vi "排气扇参数配置.vi"() -> ()   [LabVIEW 2016, in "环境动力监测库.lvlib"]
panel:
  in  "功能启用":bool
  in  "排气扇关闭温度":dbl=60.0 caption="关闭温度" format="%#_2f ℃"
  in  "排气扇开启温度":dbl=60.0 caption="开启温度" format="%#.2f ℃"
  # "排气扇参数配置"
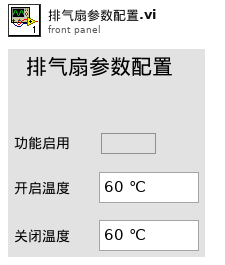
[diagram p1: front panel]
types:
  T1 = cluster{"功能启用":bool, "排气扇开启温度":dbl, "排气扇关闭温度":dbl}
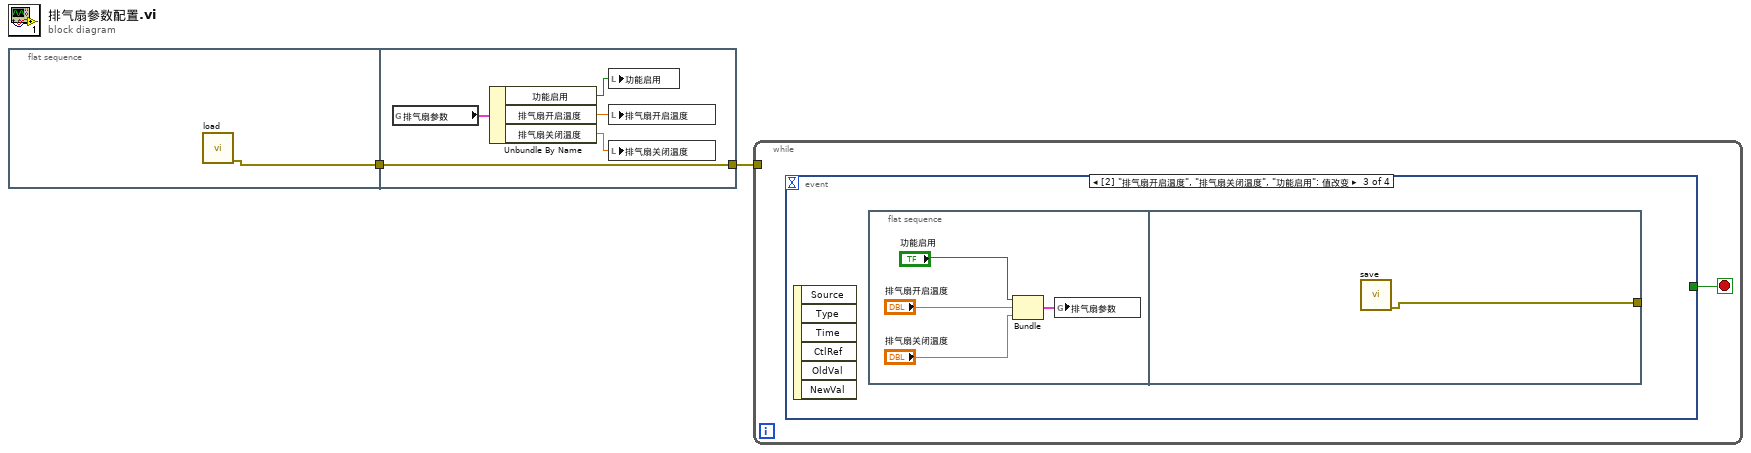
[diagram p0: block diagram]
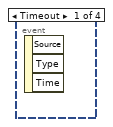
[diagram p2: hidden frame]
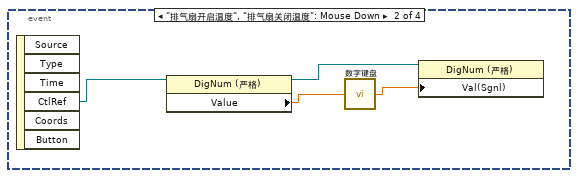
[diagram p3: hidden frame]
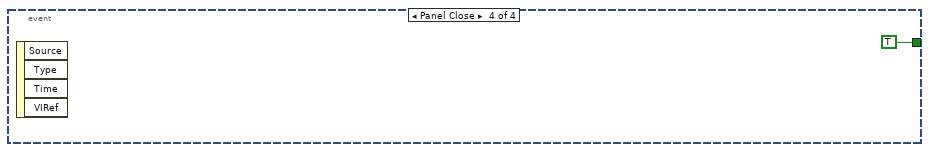
[diagram p4: hidden frame]
diagram:
  n1 = flat-sequence {
    tunnel: [w3] -> w2
    tunnel: [w8] -> w1
    tunnel: w2 -> [w8]
    frame #0 {
      n2 = call "load.vi"() -> ("error out"=w3:errorcluster)  [unwired: 11 in]
    }
    frame #1 {
      n3 = global read "断电保存全局变量.vi" "排气扇参数"() -> (w7:T1)
      n4 = Unbundle By Name(w7) -> ("功能启用"=w6:bool, "排气扇开启温度"=w5:dbl, "排气扇关闭温度"=w4:dbl)
      n5 = local write "功能启用"(w6) -> ()
      n6 = local write "排气扇开启温度"(w5) -> ()
      n7 = local write "排气扇关闭温度"(w4) -> ()
    }
  }
  n8 = while {
    tunnel: w1 -> [_]
    stop <- w9 stop-if-true
    n9 = event shown="[2] \"排气扇开启温度\", \"排气扇关闭温度\", \"功能启用\": 值改变" {
      selector: _ -> [_ _ _ _]
      dyn-events: _ -> [_ _ _ _]
      timeout: _ -> [_ _ _ _]
      tunnel: [_ _ _ TRUE] -> w9
      event Timeout {
        n10 = event-data() -> ()  [unwired: 1 in, 3 out]
      }
      event "排气扇开启温度", "排气扇关闭温度": Mouse Down {
        n11 = event-data() -> ("CtlRef"=w10:refnum<vi>)  [unwired: 1 in, 5 out]
        n12 = property class="DigNum (严格)"(reference=w10) -> (reference out=w12:refnum<vi>, "Value"=w13:dbl)  [unwired: 1 in, 1 out]
        n13 = call "数字键盘.vi"("OldNumber"=w13) -> ("NewNumber"=w11:sgl)
        n14 = property class="DigNum (严格)"(reference=w12, "Val(Sgnl)"=w11) -> ()  [unwired: 1 in, 2 out]
      }
      event "排气扇开启温度", "排气扇关闭温度", "功能启用": Value Change {
        n15 = event-data() -> ()  [unwired: 1 in, 6 out]
        n16 = flat-sequence {
          tunnel: [w18] -> _
          frame #0 {
            n17 = Bundle("功能启用"="功能启用", "排气扇开启温度"="排气扇开启温度", "排气扇关闭温度"="排气扇关闭温度") -> (w15:T1)  [unwired: 1 in]
            n18 = global write "断电保存全局变量.vi" "排气扇参数"(w15) -> ()
          }
          frame #1 {
            n19 = call "save.vi"() -> ("error out"=w18:errorcluster)  [unwired: 11 in]
          }
        }
      }
      event Panel Close {
        n20 = event-data() -> ()  [unwired: 1 in, 4 out]
      }
    }
  }
